vi "Cervena-NeniNutno.vi"(11 "NXT/EV3":T1) -> (3 "NXT/EV3 2":T1)   [LabVIEW 2016]
uses:
  <vilib>/NXT/Subs/LVHSConnector.ctl
  <vilib>/NXT/LegoClasses/BrickReference/BrickReference.lvclass
  <vilib>/NXT/Dual Mode Library/Sound/PlayG.vi
  <vilib>/NXT/Dual Mode Library/Display/drawText_Center.vi
  <vilib>/NXT/Dual Mode Library/Sound/PlayF.vi
  <vilib>/NXT/Dual Mode Library/Sound/PlayE.vi
  <vilib>/NXT/Dual Mode Library/Sound/PlayD.vi
  <vilib>/NXT/Dual Mode Library/Waits/Wait_Num.vi
  <vilib>/NXT/Dual Mode Library/Sound/PlayC.vi
  <vilib>/NXT/Dual Mode Library/Sound/PlayB.vi
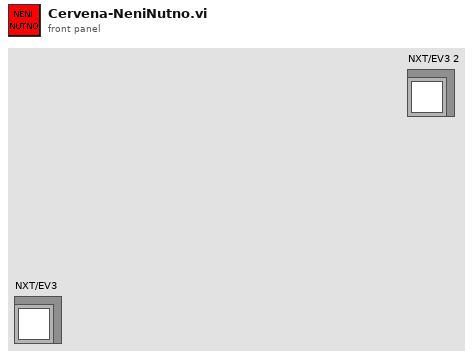
[diagram p1: front panel]
types:
  T1 = typedef "LVHSConnector.ctl" = refnum<class "BrickReference.lvclass">
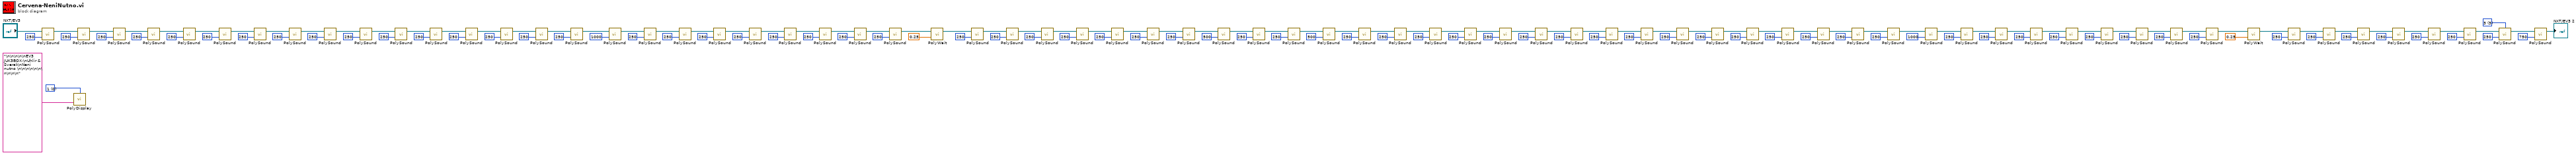
[diagram p0: block diagram]
diagram:
  w3 = u16 3 items=["3"=3, "4"=4, "5"=5, "6"=6, "7"=7] ("Octave")
  w144 = i16 0 items=["1", "2", "3", "4", "5", "6", "7", "8", "9", "10", "11", "12"] ("Line")
  n1 = call-poly <vilib>:"PolySound.vi"("Duration (500 ms)"=u16 250, "NXT/EV3"="NXT/EV3") -> ("NXT/EV3"=w140:T1)  [unwired: 2 in]
  n2 = call-poly <vilib>:"PolyDisplay.vi"("Text"="\n\n\n\n\nEV3 JUK3BOX:\nUhlir & Sverak\nNeni nutno \n\n\n\n\n\n\n\n\n\n", "Line"=w144) -> ()  [unwired: 2 in, 1 out]
  n3 = call-poly <vilib>:"PolySound.vi"("Duration (500 ms)"=u16 250, "NXT/EV3"=w140) -> ("NXT/EV3"=w139:T1)  [unwired: 2 in]
  n4 = call-poly <vilib>:"PolySound.vi"("Duration (500 ms)"=u16 250, "NXT/EV3"=w139) -> ("NXT/EV3"=w138:T1)  [unwired: 2 in]
  n5 = call-poly <vilib>:"PolySound.vi"("Duration (500 ms)"=u16 250, "NXT/EV3"=w138) -> ("NXT/EV3"=w130:T1)  [unwired: 2 in]
  n6 = call-poly <vilib>:"PolySound.vi"("Duration (500 ms)"=u16 250, "NXT/EV3"=w130) -> ("NXT/EV3"=w135:T1)  [unwired: 2 in]
  n7 = call-poly <vilib>:"PolySound.vi"("Duration (500 ms)"=u16 250, "NXT/EV3"=w135) -> ("NXT/EV3"=w136:T1)  [unwired: 2 in]
  n8 = call-poly <vilib>:"PolySound.vi"("Duration (500 ms)"=u16 250, "NXT/EV3"=w136) -> ("NXT/EV3"=w137:T1)  [unwired: 2 in]
  n9 = call-poly <vilib>:"PolySound.vi"("Duration (500 ms)"=u16 250, "NXT/EV3"=w137) -> ("NXT/EV3"=w123:T1)  [unwired: 2 in]
  n10 = call-poly <vilib>:"PolySound.vi"("Duration (500 ms)"=u16 250, "NXT/EV3"=w123) -> ("NXT/EV3"=w125:T1)  [unwired: 2 in]
  n11 = call-poly <vilib>:"PolySound.vi"("Duration (500 ms)"=u16 250, "NXT/EV3"=w125) -> ("NXT/EV3"=w124:T1)  [unwired: 2 in]
  n12 = call-poly <vilib>:"PolySound.vi"("Duration (500 ms)"=u16 250, "NXT/EV3"=w124) -> ("NXT/EV3"=w122:T1)  [unwired: 2 in]
  n13 = call-poly <vilib>:"PolySound.vi"("Duration (500 ms)"=u16 250, "NXT/EV3"=w122) -> ("NXT/EV3"=w114:T1)  [unwired: 2 in]
  n14 = call-poly <vilib>:"PolySound.vi"("Duration (500 ms)"=u16 250, "NXT/EV3"=w114) -> ("NXT/EV3"=w119:T1)  [unwired: 2 in]
  n15 = call-poly <vilib>:"PolySound.vi"("Duration (500 ms)"=u16 250, "NXT/EV3"=w119) -> ("NXT/EV3"=w120:T1)  [unwired: 2 in]
  n16 = call-poly <vilib>:"PolySound.vi"("Duration (500 ms)"=u16 250, "NXT/EV3"=w120) -> ("NXT/EV3"=w121:T1)  [unwired: 2 in]
  n17 = call-poly <vilib>:"PolySound.vi"("Duration (500 ms)"=u16 250, "NXT/EV3"=w121) -> ("NXT/EV3"=w112:T1)  [unwired: 2 in]
  n18 = call-poly <vilib>:"PolySound.vi"("Duration (500 ms)"=u16 1000, "NXT/EV3"=w112) -> ("NXT/EV3"=w104:T1)  [unwired: 2 in]
  n19 = call-poly <vilib>:"PolySound.vi"("Duration (500 ms)"=u16 250, "NXT/EV3"=w104) -> ("NXT/EV3"=w109:T1)  [unwired: 2 in]
  n20 = call-poly <vilib>:"PolySound.vi"("Duration (500 ms)"=u16 250, "NXT/EV3"=w109) -> ("NXT/EV3"=w110:T1)  [unwired: 2 in]
  n21 = call-poly <vilib>:"PolySound.vi"("Duration (500 ms)"=u16 250, "NXT/EV3"=w110) -> ("NXT/EV3"=w111:T1)  [unwired: 2 in]
  n22 = call-poly <vilib>:"PolySound.vi"("Duration (500 ms)"=u16 250, "NXT/EV3"=w111) -> ("NXT/EV3"=w96:T1)  [unwired: 2 in]
  n23 = call-poly <vilib>:"PolySound.vi"("Duration (500 ms)"=u16 250, "NXT/EV3"=w96) -> ("NXT/EV3"=w99:T1)  [unwired: 2 in]
  n24 = call-poly <vilib>:"PolySound.vi"("Duration (500 ms)"=u16 250, "NXT/EV3"=w99) -> ("NXT/EV3"=w98:T1)  [unwired: 2 in]
  n25 = call-poly <vilib>:"PolySound.vi"("Duration (500 ms)"=u16 250, "NXT/EV3"=w98) -> ("NXT/EV3"=w97:T1)  [unwired: 2 in]
  n26 = call-poly <vilib>:"PolySound.vi"("Duration (500 ms)"=u16 250, "NXT/EV3"=w97) -> ("NXT/EV3"=w94:T1)  [unwired: 2 in]
  n27 = call-poly <vilib>:"PolyWait.vi"("Time (1 sec)"=sgl 0.25, "NXT/EV3"=w94) -> ("NXT/EV3"=w80:T1)  [unwired: 2 in]
  n28 = call-poly <vilib>:"PolySound.vi"("Duration (500 ms)"=u16 250, "NXT/EV3"=w80) -> ("NXT/EV3"=w90:T1)  [unwired: 2 in]
  n29 = call-poly <vilib>:"PolySound.vi"("Duration (500 ms)"=u16 250, "NXT/EV3"=w90) -> ("NXT/EV3"=w89:T1)  [unwired: 2 in]
  n30 = call-poly <vilib>:"PolySound.vi"("Duration (500 ms)"=u16 250, "NXT/EV3"=w89) -> ("NXT/EV3"=w81:T1)  [unwired: 2 in]
  n31 = call-poly <vilib>:"PolySound.vi"("Duration (500 ms)"=u16 250, "NXT/EV3"=w81) -> ("NXT/EV3"=w86:T1)  [unwired: 2 in]
  n32 = call-poly <vilib>:"PolySound.vi"("Duration (500 ms)"=u16 250, "NXT/EV3"=w86) -> ("NXT/EV3"=w87:T1)  [unwired: 2 in]
  n33 = call-poly <vilib>:"PolySound.vi"("Duration (500 ms)"=u16 250, "NXT/EV3"=w87) -> ("NXT/EV3"=w88:T1)  [unwired: 2 in]
  n34 = call-poly <vilib>:"PolySound.vi"("Duration (500 ms)"=u16 250, "NXT/EV3"=w88) -> ("NXT/EV3"=w77:T1)  [unwired: 2 in]
  n35 = call-poly <vilib>:"PolySound.vi"("Duration (500 ms)"=u16 500, "NXT/EV3"=w77) -> ("NXT/EV3"=w74:T1)  [unwired: 2 in]
  n36 = call-poly <vilib>:"PolySound.vi"("Duration (500 ms)"=u16 250, "NXT/EV3"=w74) -> ("NXT/EV3"=w75:T1)  [unwired: 2 in]
  n37 = call-poly <vilib>:"PolySound.vi"("Duration (500 ms)"=u16 250, "NXT/EV3"=w75) -> ("NXT/EV3"=w72:T1)  [unwired: 2 in]
  n38 = call-poly <vilib>:"PolySound.vi"("Duration (500 ms)"=u16 500, "NXT/EV3"=w72) -> ("NXT/EV3"=w5:T1)  [unwired: 2 in]
  n39 = call-poly <vilib>:"PolySound.vi"("Duration (500 ms)"=u16 250, "NXT/EV3"=w5) -> ("NXT/EV3"=w10:T1)  [unwired: 2 in]
  n40 = call-poly <vilib>:"PolySound.vi"("Duration (500 ms)"=u16 250, "NXT/EV3"=w10) -> ("NXT/EV3"=w11:T1)  [unwired: 2 in]
  n41 = call-poly <vilib>:"PolySound.vi"("Duration (500 ms)"=u16 250, "NXT/EV3"=w11) -> ("NXT/EV3"=w12:T1)  [unwired: 2 in]
  n42 = call-poly <vilib>:"PolySound.vi"("Duration (500 ms)"=u16 250, "NXT/EV3"=w12) -> ("NXT/EV3"=w20:T1)  [unwired: 2 in]
  n43 = call-poly <vilib>:"PolySound.vi"("Duration (500 ms)"=u16 250, "NXT/EV3"=w20) -> ("NXT/EV3"=w15:T1)  [unwired: 2 in]
  n44 = call-poly <vilib>:"PolySound.vi"("Duration (500 ms)"=u16 250, "NXT/EV3"=w15) -> ("NXT/EV3"=w14:T1)  [unwired: 2 in]
  n45 = call-poly <vilib>:"PolySound.vi"("Duration (500 ms)"=u16 250, "NXT/EV3"=w14) -> ("NXT/EV3"=w13:T1)  [unwired: 2 in]
  n46 = call-poly <vilib>:"PolySound.vi"("Duration (500 ms)"=u16 250, "NXT/EV3"=w13) -> ("NXT/EV3"=w27:T1)  [unwired: 2 in]
  n47 = call-poly <vilib>:"PolySound.vi"("Duration (500 ms)"=u16 250, "NXT/EV3"=w27) -> ("NXT/EV3"=w25:T1)  [unwired: 2 in]
  n48 = call-poly <vilib>:"PolySound.vi"("Duration (500 ms)"=u16 250, "NXT/EV3"=w25) -> ("NXT/EV3"=w26:T1)  [unwired: 2 in]
  n49 = call-poly <vilib>:"PolySound.vi"("Duration (500 ms)"=u16 250, "NXT/EV3"=w26) -> ("NXT/EV3"=w28:T1)  [unwired: 2 in]
  n50 = call-poly <vilib>:"PolySound.vi"("Duration (500 ms)"=u16 250, "NXT/EV3"=w28) -> ("NXT/EV3"=w36:T1)  [unwired: 2 in]
  n51 = call-poly <vilib>:"PolySound.vi"("Duration (500 ms)"=u16 250, "NXT/EV3"=w36) -> ("NXT/EV3"=w31:T1)  [unwired: 2 in]
  n52 = call-poly <vilib>:"PolySound.vi"("Duration (500 ms)"=u16 250, "NXT/EV3"=w31) -> ("NXT/EV3"=w30:T1)  [unwired: 2 in]
  n53 = call-poly <vilib>:"PolySound.vi"("Duration (500 ms)"=u16 250, "NXT/EV3"=w30) -> ("NXT/EV3"=w29:T1)  [unwired: 2 in]
  n54 = call-poly <vilib>:"PolySound.vi"("Duration (500 ms)"=u16 250, "NXT/EV3"=w29) -> ("NXT/EV3"=w38:T1)  [unwired: 2 in]
  n55 = call-poly <vilib>:"PolySound.vi"("Duration (500 ms)"=u16 1000, "NXT/EV3"=w38) -> ("NXT/EV3"=w46:T1)  [unwired: 2 in]
  n56 = call-poly <vilib>:"PolySound.vi"("Duration (500 ms)"=u16 250, "NXT/EV3"=w46) -> ("NXT/EV3"=w41:T1)  [unwired: 2 in]
  n57 = call-poly <vilib>:"PolySound.vi"("Duration (500 ms)"=u16 250, "NXT/EV3"=w41) -> ("NXT/EV3"=w40:T1)  [unwired: 2 in]
  n58 = call-poly <vilib>:"PolySound.vi"("Duration (500 ms)"=u16 250, "NXT/EV3"=w40) -> ("NXT/EV3"=w39:T1)  [unwired: 2 in]
  n59 = call-poly <vilib>:"PolySound.vi"("Duration (500 ms)"=u16 250, "NXT/EV3"=w39) -> ("NXT/EV3"=w54:T1)  [unwired: 2 in]
  n60 = call-poly <vilib>:"PolySound.vi"("Duration (500 ms)"=u16 250, "NXT/EV3"=w54) -> ("NXT/EV3"=w51:T1)  [unwired: 2 in]
  n61 = call-poly <vilib>:"PolySound.vi"("Duration (500 ms)"=u16 250, "NXT/EV3"=w51) -> ("NXT/EV3"=w52:T1)  [unwired: 2 in]
  n62 = call-poly <vilib>:"PolySound.vi"("Duration (500 ms)"=u16 250, "NXT/EV3"=w52) -> ("NXT/EV3"=w53:T1)  [unwired: 2 in]
  n63 = call-poly <vilib>:"PolySound.vi"("Duration (500 ms)"=u16 250, "NXT/EV3"=w53) -> ("NXT/EV3"=w56:T1)  [unwired: 2 in]
  n64 = call-poly <vilib>:"PolyWait.vi"("Time (1 sec)"=sgl 0.25, "NXT/EV3"=w56) -> ("NXT/EV3"=w70:T1)  [unwired: 2 in]
  n65 = call-poly <vilib>:"PolySound.vi"("Duration (500 ms)"=u16 250, "NXT/EV3"=w70) -> ("NXT/EV3"=w60:T1)  [unwired: 2 in]
  n66 = call-poly <vilib>:"PolySound.vi"("Duration (500 ms)"=u16 250, "NXT/EV3"=w60) -> ("NXT/EV3"=w61:T1)  [unwired: 2 in]
  n67 = call-poly <vilib>:"PolySound.vi"("Duration (500 ms)"=u16 250, "NXT/EV3"=w61) -> ("NXT/EV3"=w69:T1)  [unwired: 2 in]
  n68 = call-poly <vilib>:"PolySound.vi"("Duration (500 ms)"=u16 250, "NXT/EV3"=w69) -> ("NXT/EV3"=w64:T1)  [unwired: 2 in]
  n69 = call-poly <vilib>:"PolySound.vi"("Duration (500 ms)"=u16 250, "NXT/EV3"=w64) -> ("NXT/EV3"=w63:T1)  [unwired: 2 in]
  n70 = call-poly <vilib>:"PolySound.vi"("Duration (500 ms)"=u16 250, "NXT/EV3"=w63) -> ("NXT/EV3"=w62:T1)  [unwired: 2 in]
  n71 = call-poly <vilib>:"PolySound.vi"("Duration (500 ms)"=u16 250, "NXT/EV3"=w62, "Octave"=w3) -> ("NXT/EV3"=w2:T1)  [unwired: 1 in]
  n72 = call-poly <vilib>:"PolySound.vi"("Duration (500 ms)"=u16 750, "NXT/EV3"=w2) -> ("NXT/EV3"=→"NXT/EV3 2":T1)  [unwired: 2 in]
